vi "AlliGator Get ROI Intensity Array v4.vi"(8 "error in (no error)":errorcluster, 10 "ROI Descriptor":T2 {"Contours"."Type" items=["No Selection", "Point", "Line", "Rectangle", "Oval", "Polygon", "Freehand Region", "Annulus", "Unused2", "Unused3", "Broken Line", "Freehand Line", "Rotated Rectangle"]}, 11 "Images":cluster{"Image Sum":T1, "Image Array":T1[]}) -> (0 "Error Out":errorcluster, 1 "# Valid Pixels":i32, 2 "# Pixels":i32, 3 "ROI Intensity Array":dbl[](array[numeric]), 4 "CPU (s)":dbl, 5 "ROI Center":cluster{"X":i32, "Y":i32})   [LabVIEW 2021, in "AlliGator Decay Processing.lvlib"]
doc: "Gets the intensity array for the provided ROI."
uses:
  AlliGator Decay Processing.lvlib
  <vilib>/vision/Image Controls.llb/IMAQ Image.ctl
  Source Image/AlliGator Source Image.lvlib
  Time/Time.lvlib
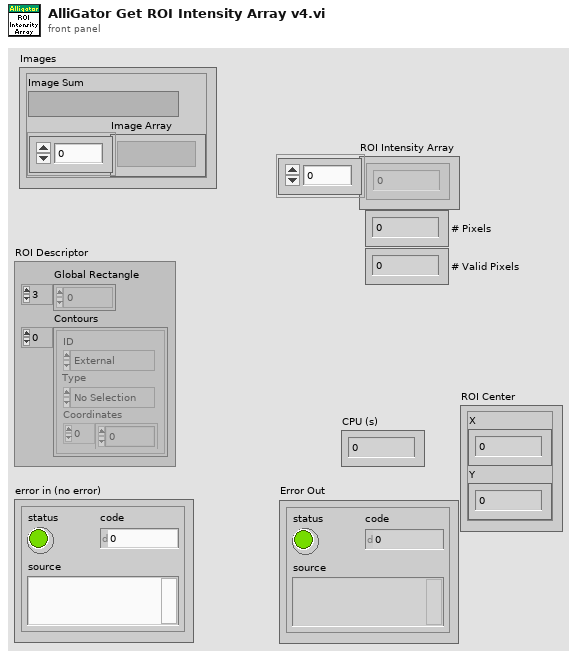
[diagram p1: front panel]
types:
  T1 = typedef "IMAQ Image.ctl" = refnum<image>
  T2 = typedef "ROI Descriptor" = cluster{"Global Rectangle":i32[], "Contours":cluster{"ID":enum32{"External", "Internal"}, "Type":u32, "Coordinates":i32[]}[]}
  T3 = typedef "AlliGator Settings.lvlib/AlliGator Pixel Counts Constraints.ctl" = cluster{"High Count Pixels Rejection Options":T4, "Low Count Pixels Rejection Options":T5}
  T4 = typedef "AlliGator Settings.lvlib/AlliGator High Count Pixels Rejection Options.ctl" = cluster{"Background High Threshold Factor":dbl, "Fixed High Background Threshold":dbl, "Reject High Count Pixels":bool, "High Percentile":dbl}
  T5 = typedef "AlliGator Settings.lvlib/AlliGator Low Count Pixels Rejection Options.ctl" = cluster{"Background Low Threshold Factor":dbl, "Fixed Low Background Threshold":dbl, "Reject Low Count Pixels":bool, "Low Percentile":dbl}
  T6 = cluster{"Decay Peak Constraint":bool, "Min":dbl, "Max":dbl}
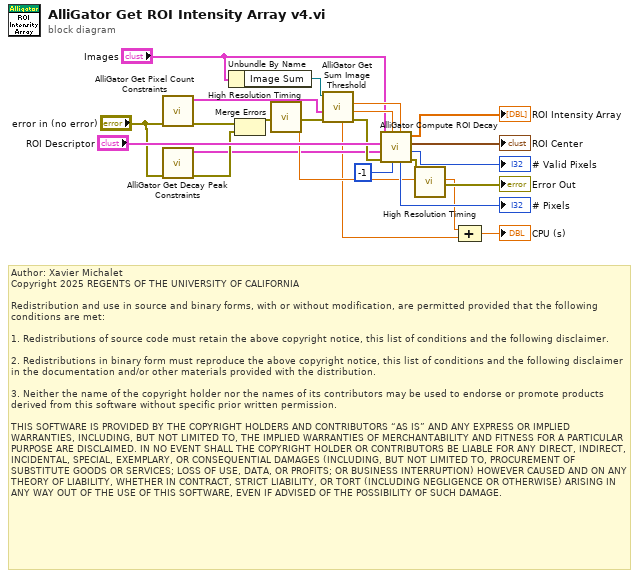
[diagram p0: block diagram]
diagram:
  # "Author: Xavier Michalet\nCopyright 2025 REGENTS OF THE UNIVERSITY OF CALIFORNIA\n\nRedistribution and use in source and binary forms, with or without modification, are permitted provided that the following conditions are met:\n\n1. Redistributions of source code must retain the above copyright notice, this list of conditions and the following disclaimer.\n\n2. Redistributions in binary form must reproduce the above copyright notice, this list of conditions and the following disclaimer in the documentation and/or other materials provided with the distribution.\n\n3. Neither the name of the copyright holder nor the names of its contributors may be used to endorse or promote products derived from this software without specific prior written permission.\n\nTHIS SOFTWARE IS PROVIDED BY THE COPYRIGHT HOLDERS AND CONTRIBUTORS “AS IS” AND ANY EXPRESS OR IMPLIED WARRANTIES, INCLUDING, BUT NOT LIMITED TO, THE IMPLIED WARRANTIES OF MERCHANTABILITY AND FITNESS FOR A PARTICULAR PURPOSE ARE DISCLAIMED. IN NO EVENT SHALL THE COPYRIGHT HOLDER OR CONTRIBUTORS BE LIABLE FOR ANY DIRECT, INDIRECT, INCIDENTAL, SPECIAL, EXEMPLARY, OR CONSEQUENTIAL DAMAGES (INCLUDING, BUT NOT LIMITED TO, PROCUREMENT OF SUBSTITUTE GOODS OR SERVICES; LOSS OF USE, DATA, OR PROFITS; OR BUSINESS INTERRUPTION) HOWEVER CAUSED AND ON ANY THEORY OF LIABILITY, WHETHER IN CONTRACT, STRICT LIABILITY, OR TORT (INCLUDING NEGLIGENCE OR OTHERWISE) ARISING IN ANY WAY OUT OF THE USE OF THIS SOFTWARE, EVEN IF ADVISED OF THE POSSIBILITY OF SUCH DAMAGE."
  n1 = call "AlliGator Get Pixel Count Constraints.vi"("error in (no error)"="error in (no error)") -> ("error out"=w24:errorcluster, "Pixel Count Constraints"=w4:T3)  [unwired: 9 in]
  n2 = call "AlliGator Get Decay Peak Constraints.vi"("error in (no error)"="error in (no error)") -> ("Error Out"=w11:errorcluster, "Decay Peak Constraints"=w5:T6)  [unwired: 9 in]
  n3 = Unbundle By Name("Images") -> ("Image Sum"=w21:T1)
  n4 = Merge Errors(w24, w11) -> (w23:errorcluster)
  n5 = call "High Resolution Timing.vi"("Error In"=w23) -> ("elapsed (relative) seconds"=w7:dbl, "Error Out"=w9:errorcluster)  [unwired: 16 in, 1 out]
  n6 = call "AlliGator Get Sum Image Threshold.vi"("error in (no error)"=w9, "Pixel Counts Constraints"=w4, "Image in"=w21) -> ("error out"=w12:errorcluster, "Pixel Threshold Low"=w14:sgl, "Pixel Threshold High"=w15:sgl, "elapsed (relative) seconds"=w2:dbl)  [unwired: 2 in, 3 out]
  n7 = call "AlliGator Compute ROI Decay.vi"("Pixel Threshold High"=w15, "Loop ID"=-1, "Pixel Threshold Low"=w14, "error in (no error)"=w12, "Decay Peak  Constraints"=w5, "ROI Descriptor"="ROI Descriptor", "Images"="Images") -> ("error out"=w22:errorcluster, "# Valid Pixels"=→"# Valid Pixels":i32, "ROI Center"=→"ROI Center":cluster{"X":i32, "Y":i32}, "Decay Points"=→"ROI Intensity Array":dbl[], "# Pixels"=→"# Pixels":i32)
  n8 = call "High Resolution Timing.vi"("relative seconds (NaN)"=w7, "Error In"=w22) -> ("elapsed (relative) seconds"=w6:dbl, "Error Out"=→"Error Out":errorcluster)  [unwired: 15 in, 1 out]
  n9 = Compound Arithmetic op=ADD(w6, w2) -> (→"CPU (s)":dbl)
